vi "InitStateQueue.vi"(7 "QueueMaxNumber":i32=-1, 8 "error in":errorcluster, 9 "States":T1=enum."TestSequence") -> (0 "error out":errorcluster, 3 "QueueOut":variant)   [LabVIEW 2013]
uses:
  Ctl/States.ctl
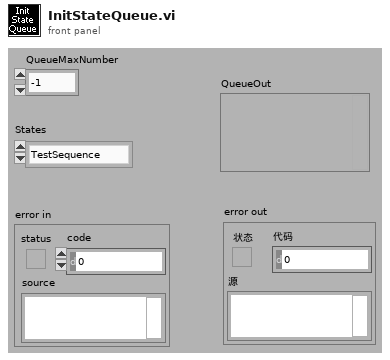
[diagram p1: front panel]
types:
  T1 = typedef "States.ctl" = enum16{"Init", "PreUUT", "Idle", "SetUp", "TestSequence", "PostUUT", "StopTest", "Debug Mode", "Selection Mode", "Loop Mode", "Error", "Wait"}
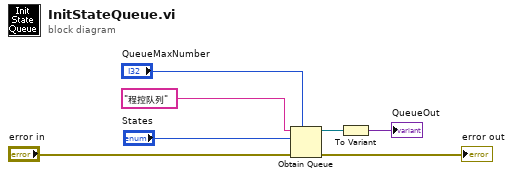
[diagram p0: block diagram]
diagram:
  n1 = Obtain Queue(max queue size (-1, unlimited)="QueueMaxNumber", name (unnamed)="程控队列" ("名称（未命名）"), element data type="States", error in (no error)="error in") -> (queue out=w6:refnum<queue>, error out=→"error out":errorcluster)  [unwired: 1 in, 1 out]
  n2 = To Variant(anything=w6) -> (Variant=→"QueueOut":variant)
